vi "AllInOne.vi"() -> ()   [LabVIEW 2013]
panel:
  out "Output Bits":bool[](array[boolean])
  in  "Input Bits":bool[](array[boolean])=[FALSE, FALSE, FALSE, TRUE, TRUE, FALSE, TRUE, TRUE]
  in  "Transmitter Properties":T1 {"Window" items=["Rectangular", "Bohman", "Parzen", "Bartlett-Hanning", "Blackman-Nuttall", "Blackman", "Hanning", "Hamming", "Welch", "Exact Blackman", "Blackman-Harris", "Triangle"]}
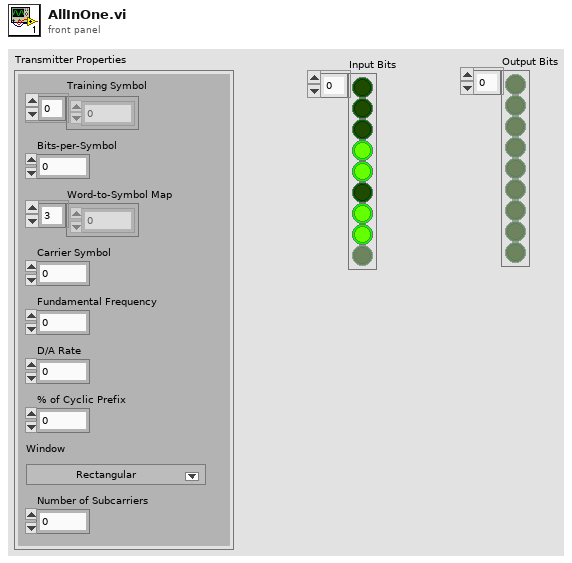
[diagram p1: front panel]
types:
  T1 = cluster{"Word-to-Symbol Map":cdb[], "% of Cyclic Prefix":dbl, "Training Symbol":cdb[], "Bits-per-Symbol":i32, "Carrier Symbol":cdb, "Fundamental Frequency":dbl, "D/A Rate":dbl, "Window":u16, "Number of Subcarriers":i32}
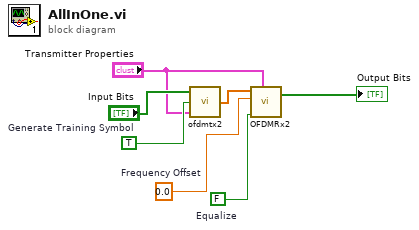
[diagram p0: block diagram]
diagram:
  w4 = 0.0  # Frequency Offset
  w5 = FALSE  # Equalize
  w7 = TRUE  # Generate Training Symbol
  n1 = call "ofdmtx2.vi"("Transmitter Properties"="Transmitter Properties", "Generate Training Symbol"=w7, "Input Bits"="Input Bits") -> ("OFDM Signal"=w3:cdb[])
  n2 = call "OFDMRx2.vi"("Input Signal"=w3, "Frequency Offset"=w4, "Equalize"=w5, "Transmitter Properties"="Transmitter Properties") -> ("Output Bits"=→"Output Bits":bool[])  [unwired: 2 in]
